vi "LIDAR_MeasureProbabilityExperiment (SubVI).vi"() -> ()   [LabVIEW 2017]
uses:
  <vilib>/Platform/TimedLoop/XDataNode/timing_clust.ctl
  <vilib>/Platform/TimedLoop/XDataNode/nitl_modes.ctl
  <vilib>/Platform/TimedLoop/XDataNode/wakeup.ctl
  Ctl/Current_Position.ctl
  <vilib>/Platform/TimedLoop/XDataNode/XDataNode.xnode
  <vilib>/Platform/TimedLoop/XDataNode/XDNodeRunTimeDep.lvlib
panel:
  out "error out":errorcluster
  in  "stop":bool
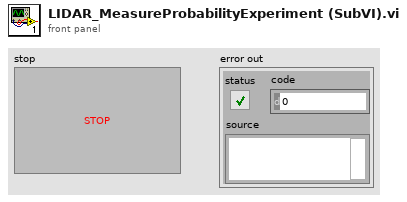
[diagram p1: front panel]
types:
  T1 = enum16{"open", "replace", "create", "open or create", "replace or create", "replace or create with confirmation"}
  T2 = typedef "_ROSControl.ctl" = cluster{"topic port":u16, "Node":string, "topic":string, "type":string, "node port":u16, "error ":errorcluster, "Direction":T3, "Update (ms)":u16, "FIFO size":u16}
  T3 = typedef "_ROSDirection.ctl" = enum16{"Node", "Publisher", "Subscriber", "ServiceClient", "ServiceProvider"}
  T4 = typedef "XDNodeRunTimeDep.lvlib/timing_clust.ctl" = cluster{"Expected End [f-1]":u64, "Actual End [f-1]":u64, "Finished Late? [f-1]":bool, "Expected End [i-1]":u64, "Actual End [i-1]":u64, "Finished Late? [i-1]":bool, "Expected Start [i]":u64, "Actual Start [i]":u64, "Expected Start [f]":u64, "Actual Start [f]":u64, "Source Name":string, "Structure Name":string, "Period":i64, "Deadline":i64, "Offset":i64, "Start":i64, "Priority":i32, "Timeout":i32, "Mode":T5, "Wakeup Reason":T6, "Error":errorcluster, "Source Type":string, "Secondary Source Type":string, "Global End Time":u64, "Global Start Time":u64, "Frame Duration":u64, "Iteration Duration":u64, "Assigned CPU":i32, "I/O Scan Engine Mode":u32}
  T5 = typedef "XDNodeRunTimeDep.lvlib/nitl_modes.ctl" = enum32{"No Change", "Process missed periods, maintain original phase", "Discard missed periods, maintain original phase", "Process missed periods, ignore original phase", "Discard missed periods, ignore original phase"}
  T6 = typedef "XDNodeRunTimeDep.lvlib/wakeup.ctl" = enum32{"Normal", "Aborted", "Asynchronous wakeup", "Timing source error", "Timed loop error", "Timeout"}
  T7 = typedef "Current_Position.ctl" = cluster{"X":dbl, "Y":dbl, "Theta":dbl}
  T8 = typedef "LaserScan.ctl" = cluster{"LaserScan_Header":cluster{"Seq":u32, "Frame ID":string, cluster{"Seconds":i32, "Nanoseconds":i32}}, "angle_min":dbl, "angle_max":dbl, "angle_increment":dbl, "time_increment":dbl, "scan_time":dbl, "range_min":dbl, "range_max":dbl, "ranges[]":dbl[], "intensities[]":dbl[]}
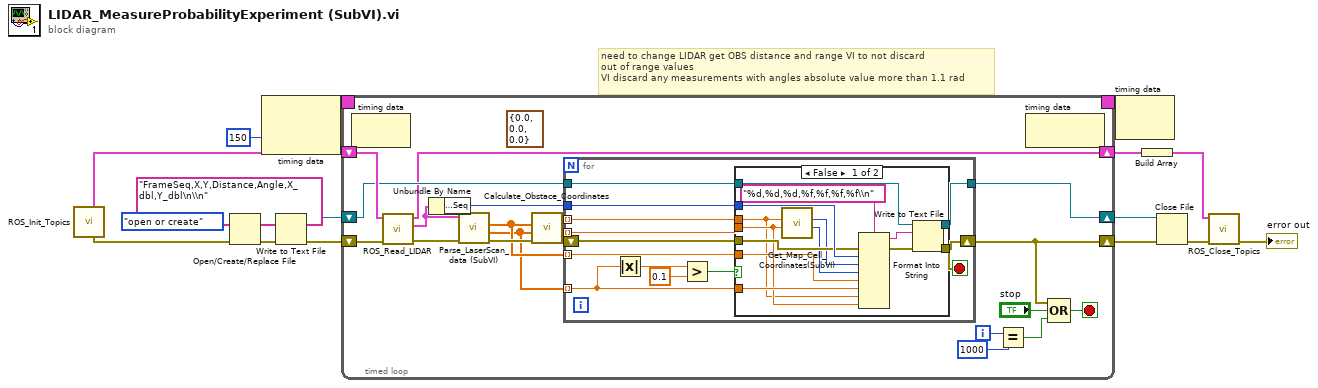
[diagram p0: block diagram]
diagram:
  # "need to change LIDAR get OBS distance and range VI to not discard \nout of range values\nVI discard any measurements with angles absolute value more than 1.1 rad"
  n1 = call "ROS_Init_Topics.vi"() -> ("error out"=w17:errorcluster, "scan_out"=w16:T2)  [unwired: 6 in, 4 out]
  n2 = Open/Create/Replace File(error in=w17, operation (0:open)=T1."open or create") -> (refnum out=w3:refnum<file>, error out=w12:errorcluster)  [unwired: 4 in, 1 out]
  n3 = node-c288(i64 150 ("Period")) -> (w15:T4)  [unwired: 1 in]
  n4 = Write to Text File(file (use dialog)=w3, text="FrameSeq,X,Y,Distance,Angle,X_dbl,Y_dbl\n\\n", error in=w12) -> (refnum out=w2:refnum<file>, error out=w4:errorcluster)  [unwired: 1 in, 1 out]
  n5 = timed-loop {
    timing: w15 -> [_]
    timing-out: [_] -> w14
    shift-right: [w22] -> w6
    shift-left: w16 -> [w36]
    shift-right: [w24] -> w10
    shift-left: w4 -> [w37]
    shift-right: [w23] -> w8
    shift-left: w2 -> [w26]
    i -> [w30]
    stop <- w32 stop-if-true
    (unwired) T7 {"X"=0.0, "Y"=0.0, "Theta"=0.0} ("Current_Position")
    n6 = node-c288() -> ()  [unwired: 1 in, 1 out]
    n7 = call "ROS_Read_LIDAR.vi"("error in (no error)"=w37, "scan_in"=w36) -> ("error out"=w35:errorcluster, "LaserScan_msg"=w20:T8, "scan_out"=w22:T2)  [unwired: 6 in, 1 out]
    n8 = Unbundle By Name(w20) -> ("LaserScan_Header.Seq"=w27:u32)
    n9 = call "Parse_LaserScan_data (SubVI).vi"("error in (no error)"=w35, "LaserScan"=w20) -> ("error in (no error) 2"=w21:errorcluster, "angles[]"=w18:dbl[], "distance[]"=w19:dbl[])  [unwired: 6 in, 1 out]
    n10 = call "Calculate_Obstace_Coordinates.vi"("error in (no error)"=w21, "angles[]"=w18, "distance[]"=w19) -> ("error out"=w25:errorcluster, "Y Out"=w33:dbl[], "X Out"=w34:dbl[])  [unwired: 5 in, 1 out]
    n11 = for {
      tunnel: w34 -> [w49] mode=indexing
      tunnel: w33 -> [w48] mode=indexing
      tunnel: w27 -> [w47]
      tunnel: w26 -> [w46]
      shift-right: [w43] -> w24
      shift-left: w25 -> [w45]
      tunnel: [w44] -> w23
      tunnel: w19 -> [w42] mode=indexing
      tunnel: w18 -> [w40] mode=indexing
      stop <- w43 stop-if-true
      n12 = Absolute Value(x=w40) -> (abs(x)=w38:dbl)
      n13 = Greater?(x=w38, y=0.1) -> (0:w41:bool)
      n14 = case shown="False" w41 {
        tunnel: w49 -> [w50 _]
        tunnel: w48 -> [w53 _]
        tunnel: w47 -> [w62 _]
        tunnel: w46 -> [w61 w64]
        tunnel: w45 -> [w54 w65]
        tunnel: [w59 w64] -> w44
        tunnel: [w57 w65] -> w43
        tunnel: w42 -> [w56 _]
        tunnel: w40 -> [w55 _]
        frame False {
          n15 = call "Get_Map_Cell_Coordinates(SubVI).vi"("Y"=w53, "X"=w50) -> ("Y_map"=w52:i32, "X_map"=w51:i32)  [unwired: 7 in, 1 out]
          n16 = Format Into String(format string="%d,%d,%d,%f,%f,%f,%f\\n", error in=w54, w62, w51, w52, w56, w55, w50, w53) -> (resulting string=w60:string, error out=w63:errorcluster)  [unwired: 1 in]
          n17 = Write to Text File(file (use dialog)=w61, text=w60, error in=w63) -> (refnum out=w59:refnum<file>, error out=w57:errorcluster)  [unwired: 1 in, 1 out]
        }
        frame True {
        }
      }
    }
    n18 = Equal?(x=w30, y=1000) -> (x = y?=w28:bool)
    n19 = node-c288() -> ()  [unwired: 1 in, 1 out]
    n20 = Compound Arithmetic op=OR(w24, "stop", w28) -> (w32:bool)
  }
  n21 = node-c288(w14) -> ()  [unwired: 1 out]
  n22 = Build Array(w6) -> (w5:T2[])
  n23 = Close File(refnum=w8, error in=w10) -> (error out=w9:errorcluster)  [unwired: 1 out]
  n24 = call "ROS_Close_Topics.vi"("error in (no error)"=w9, "ROS_In_Array"=w5) -> ("error out"=→"error out":errorcluster)  [unwired: 9 in]
